vi "GUI_Cameras_v1.2.1.vi"() -> ()   [LabVIEW 2011]
uses:
  <vilib>/Utility/miscctls.llb/LVRectTypeDef.ctl
  <vilib>/vision/NI_Vision_Development_Module.lvlib
panel:
  out "resize":bool
  in  "Tab Control":T1(tab)
  in  "analysis":bool
  out "MaxCounts":dbl(slide) scale=0.0..256.0
  in  "triggerdelay":dbl
  in  "trigger":bool
  in  "save":bool
  in  "exposure":dbl=0.52 caption="Exposure"
  in  "gain":dbl
  in  "shotnumber":i32=354
  out "Centroid":cluster{"X Centroid":sgl, "Y Centroid":sgl} {"Y Centroid" format="%.2f"; "X Centroid" format="%.2f"}
  out "Mean Value":sgl format="%.2f"
  out "Mean Value 2":sgl(graph)
  out "histogram":T2(graph)
  out "lineout":cluster{"x0":sgl, "dx":sgl, "Pixels Line":sgl[]}(graph)
  out "analysis error":errorcluster
  out "top":i16
  out "left":i16
  out "Zoom changed":bool
  out "Zoom old":cluster{"X":sgl, "Y":sgl}
  out "ratio(h)":bool=TRUE
  out "fixsize":bool
  out "Change Ratio":cluster{"X":sgl, "Y":sgl}={"X"=1.6671598, "Y"=0.6151203}
  out "old Panel Bounds":T3={"Left"=105, "Top"=80, "Right"=781, "Bottom"=662}
  out "error (h)":bool
  in  "Main Tap":enum32{"IMAQ", "Network", "Internal", "Array"}(tab)
  out "Image (IMAQ)":T4(plugin-control)
  out "local Port":u16=65401
  out "Remote Host":string="192.168.10.157"
  out "port or service name":u16=65400
  in  "timeout ms (slow resp)":i32=500
  in  "reset":bool
  out "All Devices (h)":string[](array[string])
  out "centroidy":dbl
  out "fast ID (h)":refnum<k16>
  out "slow ID (h)":refnum<k16>
  out "error out":errorcluster
  out "connections (hidden)":variant[](array[variant])=[variant(refnum<k16> refnum), variant(refnum<k16> refnum)]
  in  "time to wait (main loop)":i32=200
  in  "time to wait (TCP)":i32=10
  out "Data String":string="exposure,0.520000\r\ntrigger,off\r\nsave,off\r\ngain,0.000000\r\n"
  in  "send":bool
  in  "localsavingpath":path
  out "centroidy":dbl
  out "Image (array)":u8[][](graph)
  out "Device Name (h)":string="FakeCam1"
  out "stop":bool
  out "error message":string
  out "image connection":bool
  out "data connection ok":bool
  # "Data"
  # "Image"
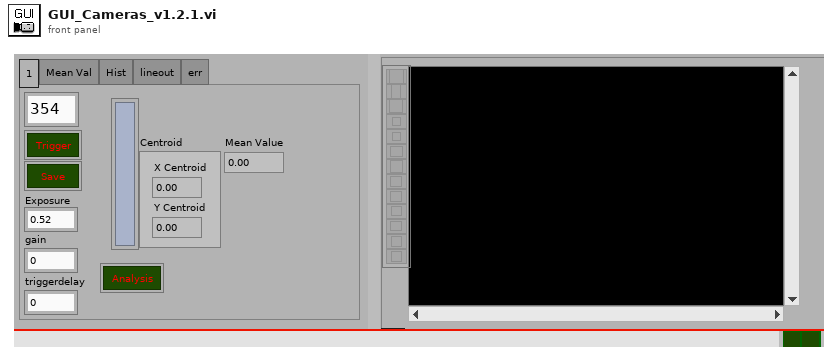
[diagram p1: front panel]
types:
  T1 = enum32{"1", "Mean Val", "Hist", "lineout", "err"}
  T2 = cluster{"Starting Value":sgl, "Incremental Value":sgl, "Histogram":u32[]}
  T3 = typedef "LVRectTypeDef.ctl" = cluster{"Left":i16, "Top":i16, "Right":i16, "Bottom":i16}
  T4 = typedef "IMAQ Image.ctl" = refnum<image>
  T5 = enum16{"Grayscale", "Binary", "Gradient", "Rainbow", "Temperature", "User Defined"}
  T6 = typedef "Image Type" = u32
  T7 = typedef "EventTypDef.ctl" = refnum<user-event>
  T8 = cluster{"Global Rectangle":i32[], "Contours":cluster{"Contour Type":u32, "ROI Type":u32, "Points":i32[]}[]}
  T9 = typedef "IMAQ Line" = cluster{"Start X":i32, "Start Y":i32, "End X":i32, "End Y":i32}
  T10 = typedef "ROI Descriptor" = cluster{"Global Rectangle":i32[], "Contours":cluster{"ID":enum32{"External", "Internal"}, "Type":u32, "Coordinates":i32[]}[]}
  T11 = typedef "LVBoundsTypeDef.ctl" = cluster{"Width":u32, "Height":u32}
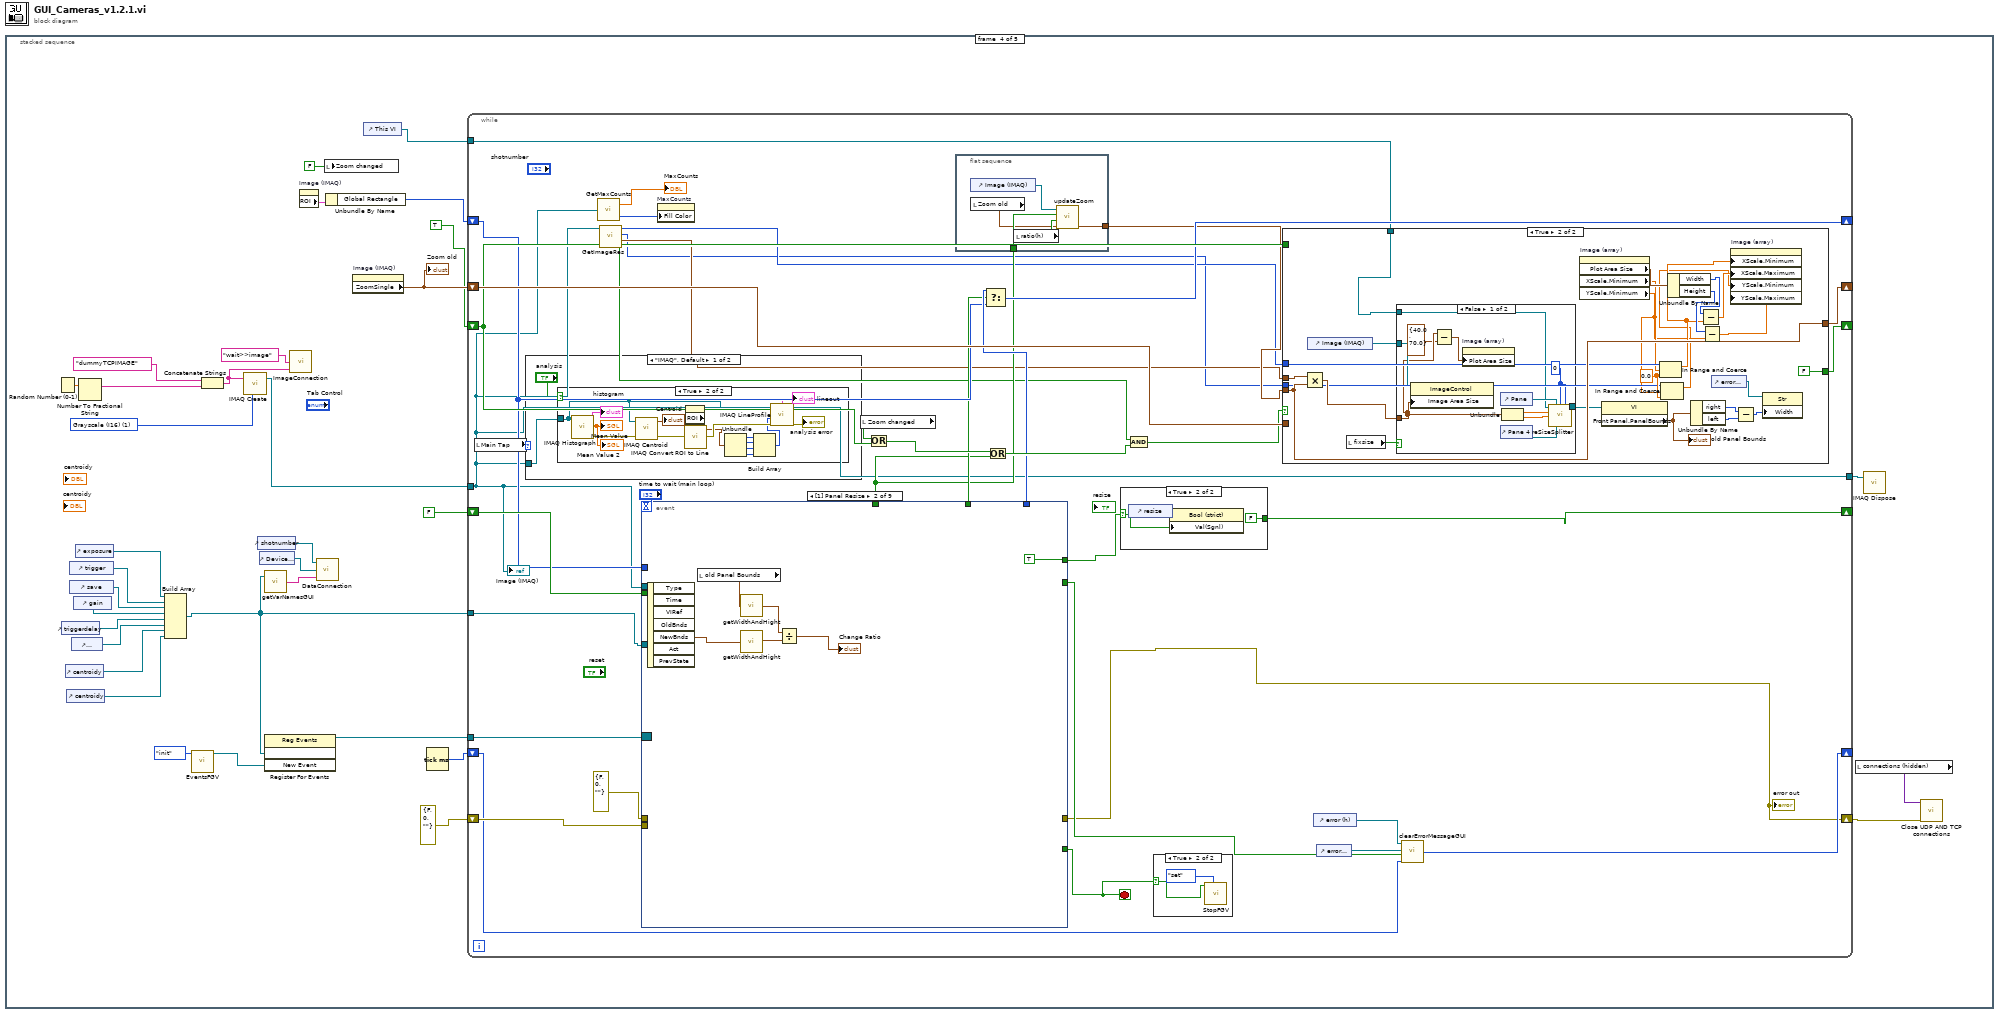
[diagram p0: block diagram]
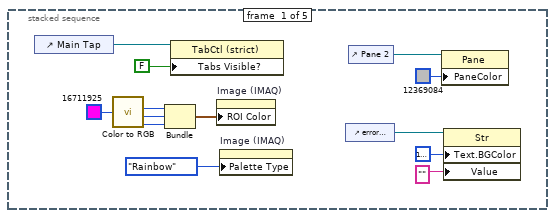
[diagram p2: hidden frame]
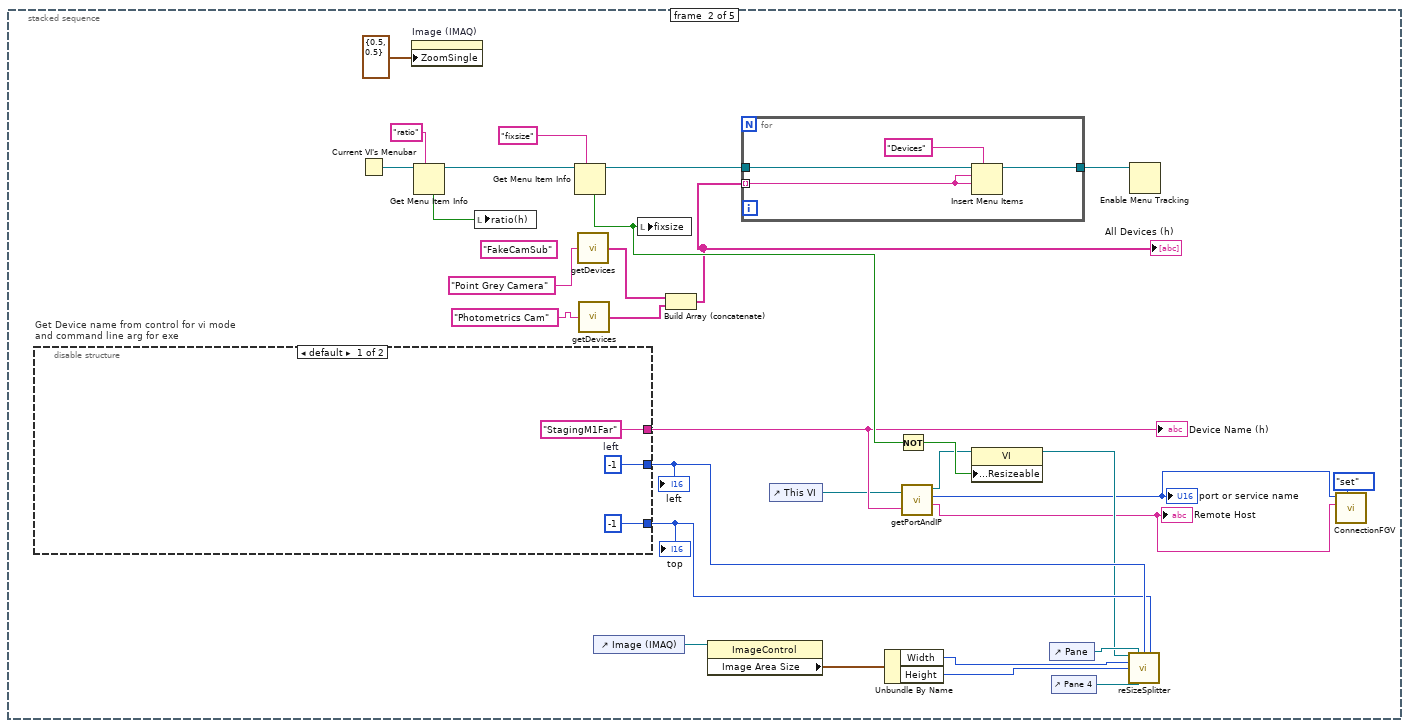
[diagram p3: hidden frame]
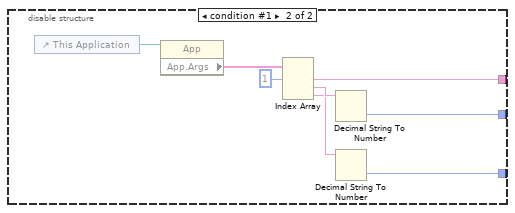
[diagram p4: hidden frame]
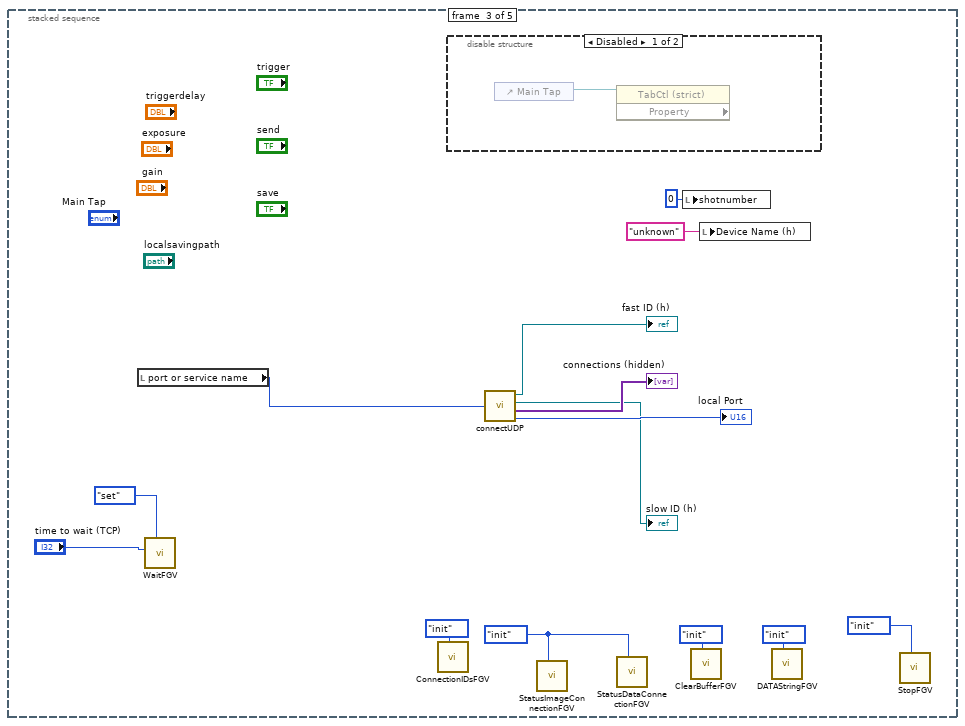
[diagram p5: hidden frame]
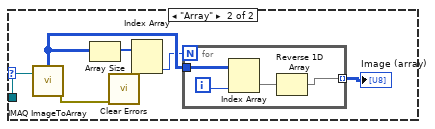
[diagram p10: hidden frame]
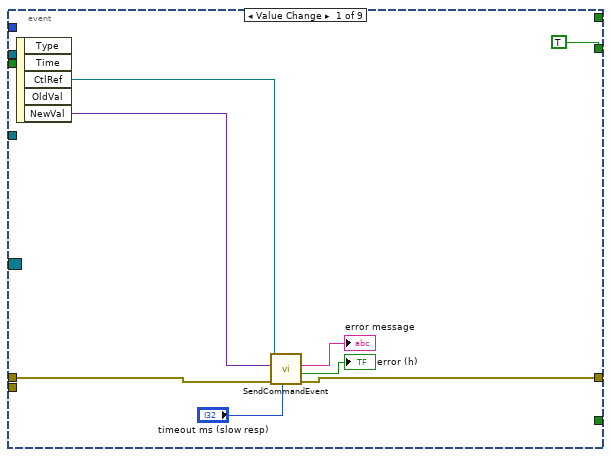
[diagram p13: hidden frame]
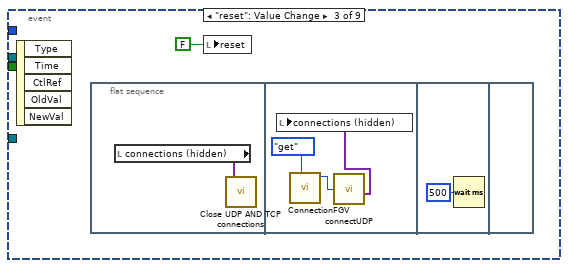
[diagram p14: hidden frame]
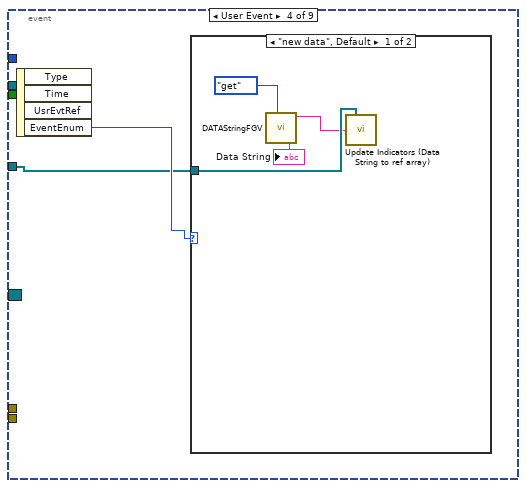
[diagram p15: hidden frame]
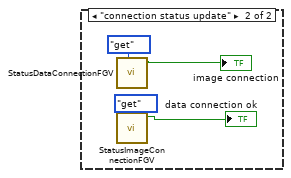
[diagram p16: hidden frame]
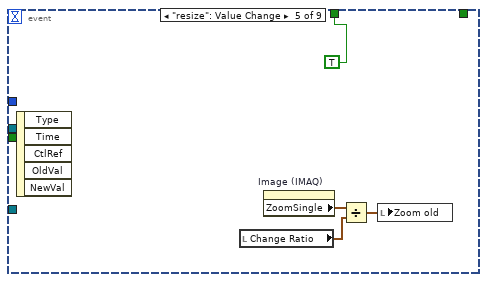
[diagram p17: hidden frame]
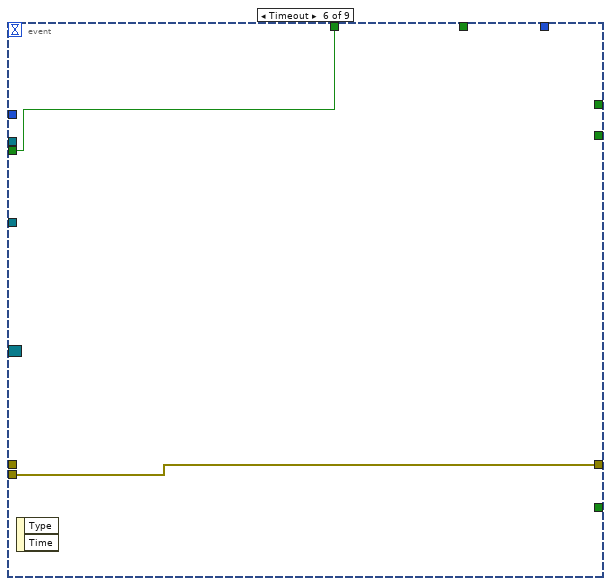
[diagram p18: hidden frame]
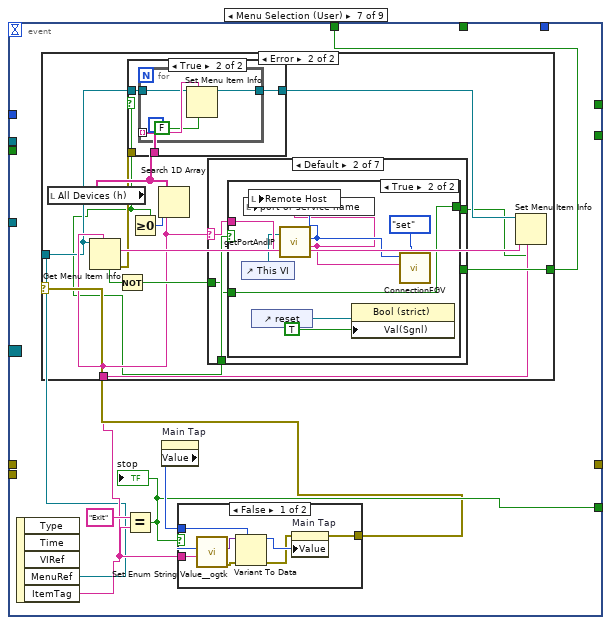
[diagram p19: hidden frame]
diagram:
  n1 = stacked-sequence {
    frame #0 {
      n2 = control-ref of="Main Tap"() -> (w13:refnum<vi>)
      n3 = call <vilib>:"Color to RGB.vi"("Color"=u32 16711925) -> ("R"=w4:u8, "G"=w3:u8, "B"=w2:u8)  [unwired: 1 out]
      n4 = Bundle("R"=w4, "G"=w3, "B"=w2) -> (w1:cluster{"R":u8, "G":u8, "B":u8})  [unwired: 1 in]
      n5 = property class="TabCtl (strict)"(reference=w13, "Tabs Visible?"=FALSE) -> ()  [unwired: 1 in, 2 out]
      n6 = property on="Image (IMAQ)" class="ImageControl"("ROI Color"=w1) -> ()  [unwired: 2 in, 2 out]
      n7 = property on="Image (IMAQ)" class="ImageControl"("Palette Type"=T5."Rainbow" ("Palette:Palette Type")) -> ()  [unwired: 2 in, 2 out]
      n8 = control-ref of="error message"() -> (w10:refnum<vi>)
      n9 = control-ref of="Pane 2"() -> (w8:refnum<vi>)
      n10 = property class="Pane"(reference=w8, "PaneColor"=u32 12369084) -> ()  [unwired: 1 in, 2 out]
      n11 = property class="Str"(reference=w10, "Text.BGColor"=u32 16777238, "Value"="") -> ()  [unwired: 1 in, 2 out]
    }
    frame #1 {
      (unwired) "FakeCamSub" ("Device Class")
      n12 = disable-structure "Get Device name from control for vi mode\nand command line arg for exe" shown="default" {
        disable-tunnel: ["StagingM1Far" ("Device Name for vi mode") w55] -> w25
        disable-tunnel: [w49 w52] -> w32
        disable-tunnel: [i16 -1 ("left") w51] -> w31
        frame condition #0 (active) {
          w49 = i16 -1  # left
        }
        frame condition #1 {
          n13 = control-ref of="This Application"() -> (w58:refnum<vi>)
          n14 = property class="App"(reference=w58) -> ("App.Args"=w57:string[])  [unwired: 1 in, 2 out]
          n15 = Index Array(array=w57, index #1=1 ("index")) -> (element #1=w55:string, element #2=w54:string, element #3=w53:string)  [unwired: 2 in]
          n16 = Decimal String To Number(string=w54) -> (number=w52:i32)  [unwired: 2 in, 1 out]
          n17 = Decimal String To Number(string=w53) -> (number=w51:i32)  [unwired: 2 in, 1 out]
        }
      }
      "Device Name (h)" <- w25
      "left" <- w32
      "top" <- w31
      n18 = Current VI's Menubar() -> (w36:refnum<k9>)
      n19 = property on="Image (IMAQ)" class="ImageControl"("ZoomSingle"=cluster{"X":sgl, "Y":sgl} {"X"=0.5, "Y"=0.5} ("ZoomSingle:All Elements")) -> ()  [unwired: 2 in, 2 out]
      n20 = Get Menu Item Info(7:"ratio" ("item tag"), 11:w36) -> (3:w34:refnum<k9>, 4:w35:bool)  [unwired: 1 in, 5 out]
      n21 = local write "ratio(h)"(w35) -> ()
      n22 = Get Menu Item Info(7:"fixsize" ("item tag"), 11:w34) -> (3:w27:refnum<k9>, 4:w29:bool)  [unwired: 1 in, 5 out]
      n23 = call "getDevices.vi"("Device Class"="Point Grey Camera") -> ("All Devices"=w16:string[])
      n24 = call "getDevices.vi"("Device Class"="Photometrics Cam") -> ("All Devices"=w15:string[])
      n25 = control-ref of="Image (IMAQ)"() -> (w43:refnum<vi>)
      n26 = local write "fixsize"(w29) -> ()
      n27 = Build Array (concatenate)(w16, w15) -> (w14:string[])
      "All Devices (h)" <- w14
      n28 = property class="ImageControl"(reference=w43) -> ("Image Area Size"=w42:cluster{"Width":u32, "Height":u32})  [unwired: 1 in, 2 out]
      n29 = for {
        tunnel: w27 -> [w47]
        tunnel: [w46] -> w26
        tunnel: w14 -> [w44] mode=indexing
        n30 = Insert Menu Items(5:"Devices" ("menu tag"), 7:w44, 8:w44, 9:w47) -> (3:w46:refnum<k9>)  [unwired: 2 in, 2 out]
      }
      n31 = control-ref of="This VI"() -> (w24:refnum<vi>)
      n32 = Unbundle By Name(w42) -> ("Width"=w41:u32, "Height"=w40:u32)
      n33 = Not(x=w29) -> (.not. x?=w30:bool)
      n34 = call "getPortAndIP.vi"("This Vi"=w24, "Device Name"=w25) -> ("reference out"=w23:refnum<vi>, "port or service name"=w20:u16, "Remote Host"=w19:string)  [unwired: 1 in]
      "port or service name" <- w20
      "Remote Host" <- w19
      n35 = property class="VI"(reference=w23, "Front Panel.Resizeable"=w30) -> (reference out=w22:refnum<vi>)  [unwired: 1 in, 1 out]
      n36 = control-ref of="Pane"() -> (w39:refnum<vi>)
      n37 = control-ref of="Pane 4"() -> (w28:refnum<vi>)
      n38 = call "reSizeSplitter.vi"("this vi"=w22, "pane"=w39, "left"=w32, "top"=w31, "Width"=w41, "Height"=w40, "pane2"=w28) -> ()  [unwired: 8 in, 1 out]
      n39 = Enable Menu Tracking(4:w26) -> ()  [unwired: 2 in, 2 out]
      n40 = call "ConnectionFGV.vi"("command"=enum16{"get", "set", "init"}."set", "Remote Host in"=w19, "port or service name in"=w20) -> ()  [unwired: 7 in, 2 out]
    }
    frame #2 {
      w68 = enum16{"get", "set", "init"}."init" ("Command")
      n41 = local read "port or service name"() -> (w70:u16)
      n42 = call "WaitFGV.vi"("Command"=enum16{"get", "set", "init"}."set", "milliseconds to wait"="time to wait (TCP)") -> ()  [unwired: 9 in, 1 out]
      n43 = call "ConnectionIDsFGV.vi"("Command"=enum16{"add", "get", "init"}."init") -> ()  [unwired: 10 in, 1 out]
      n44 = disable-structure shown="Disabled" {
        frame Disabled {
          n45 = control-ref of="Main Tap"() -> (w73:refnum<vi>)
          n46 = property class="TabCtl (strict)" props=[](reference=w73) -> ()  [unwired: 1 in, 3 out]
        }
        frame Enabled {
        }
      }
      n47 = call "connectUDP.vi"("port or service name"=w70) -> ("fast ID (h)"=→"fast ID (h)":refnum<k16>, "slow ID (h)"=→"slow ID (h)":refnum<k16>, "connections (hidden)"=→"connections (hidden)":variant[], "local Port"=→"local Port":u16)
      n48 = call "StatusImageConnectionFGV.vi"("Command"=w68) -> ()  [unwired: 10 in, 1 out]
      n49 = call "StatusDataConnectionFGV.vi"("Command"=w68) -> ()  [unwired: 10 in, 1 out]
      n50 = local write "shotnumber"(0 ("shotnumber")) -> ()
      n51 = call "ClearBufferFGV.vi"("Command"=enum16{"set", "get", "init"}."init") -> ()  [unwired: 10 in, 1 out]
      n52 = local write "Device Name (h)"("unknown" ("Device Name")) -> ()
      n53 = call "DATAStringFGV.vi"("Command"=enum16{"get", "set", "init"}."init") -> ()  [unwired: 10 in, 1 out]
      n54 = call "StopFGV.vi"("Command"=enum16{"set", "get", "init"}."init") -> ()  [unwired: 10 in, 1 out]
    }
    frame #3 {
      w105 = T6 1 items=["Grayscale (U8)", "Grayscale (I16)", "Grayscale (SGL)", "Complex (CSG)", "RGB (U32)", "HSL (U32)", "RGB (U64)", "Grayscale (U16)"] ("Image Type")
      n55 = Random Number (0-1)() -> (number: 0 to 1=w102:dbl)
      n56 = control-ref of="triggerdelay"() -> (w92:refnum<vi>)
      n57 = control-ref of="centroidy"() -> (w86:refnum<vi>)
      n58 = control-ref of="centroidy"() -> (w79:refnum<vi>)
      n59 = control-ref of="trigger"() -> (w96:refnum<vi>)
      n60 = control-ref of="save"() -> (w94:refnum<vi>)
      n61 = control-ref of="localsavingpath"() -> (w87:refnum<vi>)
      n62 = control-ref of="gain"() -> (w93:refnum<vi>)
      n63 = control-ref of="exposure"() -> (w95:refnum<vi>)
      n64 = Number To Fractional String(number=w102) -> (F-format string=w101:string)  [unwired: 3 in]
      n65 = Build Array(w95, w96, w94, w93, w92, w87, w86, w79) -> (w77:refnum<vi>[])
      n66 = call "EventsFGV.vi"("Command"=enum16{"get", "init"}."init") -> ("New Event"=w74:T7)  [unwired: 10 in]
      n67 = Concatenate Strings("dummyTCPIMAGE" ("Image Name"), w101) -> (w99:string)
      n68 = call "IMAQ Create"("Image Name"=w99, "Image Type"=w105) -> ("New Image"=w104:T4)  [unwired: 3 in, 1 out]
      n69 = control-ref of="shotnumber"() -> (w81:refnum<vi>)
      n70 = control-ref of="Device Name (h)"() -> (w80:refnum<vi>)
      n71 = call "getVarNamesGUI.vi"("Array"=w77) -> ("String"=w76:string)  [unwired: 1 in]
      n72 = register-events(w77, w74) -> (reference out=w78:refnum<event-registration>)  [unwired: 2 in, 1 out]
      n73 = call "ImageConnection.vi"("Image Name"=w99, "Image Subscriber list"="wait>>image") -> ()  [unwired: 2 in]
      n74 = property on="Image (IMAQ)" class="ImageControl"() -> ("ROI"=w85:T8)  [unwired: 2 in, 2 out]
      n75 = call "DataConnection.vi"("Subscriber list"=w76, "Device Name (h)"=w80, "shotnumber"=w81) -> ()
      n76 = local write "Zoom changed"(FALSE ("Zoom changed")) -> ()
      n77 = Unbundle By Name(w85) -> ("Global Rectangle"=w84:i32[])
      n78 = property on="Image (IMAQ)" class="ImageControl"() -> ("ZoomSingle"=w91:cluster{"X":sgl, "Y":sgl})  [unwired: 2 in, 2 out]
      "Zoom old" <- w91
      n79 = control-ref of="This VI"() -> (w83:refnum<vi>)
      n80 = Tick Count (ms)() -> (millisecond timer value=w88:u32)
      n81 = while {
        shift-right: [w110] -> w103
        shift-left: errorcluster {"status"=FALSE, "code"=0, "source"=""} ("error out") -> [w143]
        tunnel: w104 -> [w119]
        tunnel: [w119] -> w106
        tunnel: w77 -> [w111]
        shift-right: [w142] -> _
        shift-left: w91 -> [w141]
        shift-right: [w108] -> _
        shift-left: FALSE -> [w140]
        shift-right: [w139] -> _
        shift-left: TRUE -> [w138]
        shift-right: [w134] -> _
        shift-left: w88 -> [w133]
        shift-right: [w128] -> _
        shift-left: w84 -> [w127]
        tunnel: w83 -> [w125]
        tunnel: w78 -> [w112]
        stop <- w113 stop-if-true
        n82 = local read "Main Tap"() -> (w130:enum32{"IMAQ", "Network", "Internal", "Array"})
        n83 = case shown="\"IMAQ\", Default" w130 {
          tunnel: w119 -> [w158 w179]
          frame "IMAQ", Default {
            n84 = case shown="True" "analysis" {
              tunnel: w158 -> [_ w169]
              frame False {
              }
              frame True {
                n85 = call "IMAQ Histograph"("Image"=w169) -> ("error out"=w171:errorcluster, "Mean Value"=→"Mean Value" →"Mean Value 2":sgl, "Histogram Graph"=→"histogram":T2)  [unwired: 7 in, 1 out]
                n86 = call "IMAQ Centroid"("error in (no error)"=w171, "Image"=w169) -> ("error out"=w168:errorcluster, "Centroid"=→"Centroid":cluster{"X Centroid":sgl, "Y Centroid":sgl})  [unwired: 2 in]
                n87 = property on="Image (IMAQ)" class="ImageControl"() -> ("ROI"=w165:T8)  [unwired: 2 in, 2 out]
                n88 = call "IMAQ Convert ROI to Line"("ROI Descriptor"=w165) -> ("Line"=w164:T9)  [unwired: 8 in, 1 out]
                n89 = Unbundle(w164) -> ("Start X"=w163:i32, "Start Y"=w162:i32, "End X"=w161:i32, "End Y"=w160:i32)
                n90 = Build Array(w163, w162, w161, w160) -> (w159:i32[])
                n91 = call "IMAQ LineProfile"("error in (no error)"=w168, "Line Coordinates"=w159, "Image"=w169) -> ("error out"=→"analysis error":errorcluster, "Line Graph"=→"lineout":cluster{"x0":sgl, "dx":sgl, "Pixels Line":sgl[]})  [unwired: 2 in, 2 out]
              }
            }
          }
          frame "Array" {
            n92 = call "IMAQ ImageToArray"("Image"=w179) -> ("error out"=w178:errorcluster, "Image Pixels (U8)"=w175:u8[][])  [unwired: 3 in, 3 out]
            n93 = Array Size(array=w175) -> (size(s)=w177:i32[])
            n94 = call <vilib>:"Clear Errors.vi"("error in (no error)"=w178) -> ()  [unwired: 6 in, 1 out]
            n95 = Index Array(array=w177) -> (element #2=w174:i32)  [unwired: 2 in, 1 out]
            n96 = for {
              N: w174 -> [_]
              tunnel: w175 -> [w183]
              tunnel: [w181] -> w176 mode=indexing
              i -> [w180]
              n97 = Index Array(array=w183, index (col)=w180) -> (element=w182:u8[])  [unwired: 1 in]
              n98 = Reverse 1D Array(array=w182) -> (reversed array=w181:u8[])
            }
            "Image (array)" <- w176
          }
        }
        n99 = call "GetMaxCounts.vi"("New Image"=w119) -> ("Maximal Value"=→"MaxCounts":sgl, "Color"=w121:u32)
        n100 = call "GetImageRes.vi"("Image"=w119) -> ("valid Image"=w117:bool, "Image Area:Size:All Elements"=w118:cluster{"Width":u32, "Height":u32}, "Y Resolution"=w115:i32, "X Resolution"=w116:i32)  [unwired: 7 in]
        n101 = event shown="[1] Panel Resize" {
          selector: w112 -> [_ _ _ _ _ _ _ _ _]
          dyn-events: _ -> [_ _ _ _ _ _ _ _ _]
          timeout: "time to wait (main loop)" -> [_ _ _ _ _ _ _ _ _]
          tunnel: [w228 _ _ _ _ w257 _ _ _] -> w110
          tunnel: errorcluster {"status"=FALSE, "code"=0, "source"=""} ("error out") -> [w230 _ _ _ _ _ _ _ _]
          tunnel: w143 -> [_ _ _ _ _ w257 _ _ _]
          tunnel: [TRUE _ _ _ _ _ _ _ _] -> w131
          tunnel: [_ _ _ _ _ _ w262 _ _] -> w113
          tunnel: [_ _ _ _ TRUE w256 w259 _ _] -> w124
          tunnel: w140 -> [_ _ _ _ _ w256 _ _ _]
          tunnel: [_ TRUE _ _ _ _ _ _ _] -> w109
          tunnel: [_ _ _ _ _ _ _ _ w340] -> w129
          tunnel: w127 -> [_ _ _ _ _ _ _ _ w341]
          tunnel: [_ _ _ _ _ _ _ _ w334] -> w126
          tunnel: w119 -> [_ _ _ _ _ _ _ _ w343]
          tunnel: w111 -> [_ _ _ w243 _ _ _ _ _]
          event Value Change {
            n102 = event-data() -> ("CtlRef"=w225:refnum<vi>, "NewVal"=w224:variant)  [unwired: 1 in, 3 out]
            n103 = call "SendCommandEvent.vi"("timeout ms (slow resp)"="timeout ms (slow resp)", "error out 2"=w230, "NewVal"=w224, "CtlRef"=w225) -> ("error out"=w228:errorcluster, "error (h)"=→"error (h)":bool, "error message"=→"error message":string)  [unwired: 4 in, 1 out]
          }
          event Panel Resize {
            n104 = event-data() -> ("NewBnds"=w236:T3)  [unwired: 1 in, 6 out]
            n105 = local read "old Panel Bounds"() -> (w234:T3)
            n106 = call "getWidthAndHight.vi"("OldBnds"=w234) -> ("output cluster"=w233:cluster{"X":sgl, "Y":sgl})
            n107 = call "getWidthAndHight.vi"("OldBnds"=w236) -> ("output cluster"=w232:cluster{"X":sgl, "Y":sgl})
            n108 = Divide(x=w233, y=w232) -> (x/y=→"Change Ratio":cluster{"X":sgl, "Y":sgl})
          }
          event "reset": Value Change {
            n109 = event-data() -> ()  [unwired: 1 in, 5 out]
            n110 = flat-sequence {
              frame #0 {
                n111 = local read "connections (hidden)"() -> (w238:variant[])
                n112 = call "Close UDP AND TCP connections.vi"("appended array"=w238) -> ()  [unwired: 7 in]
              }
              frame #1 {
                n113 = call "ConnectionFGV.vi"("command"=enum16{"get", "set", "init"}."get") -> ("port or service name out"=w240:u16)  [unwired: 9 in, 1 out]
                n114 = call "connectUDP.vi"("port or service name"=w240) -> ("connections (hidden)"=w239:variant[])  [unwired: 3 out]
                n115 = local write "connections (hidden)"(w239) -> ()
              }
              frame #2 {
                n116 = Wait (ms)(milliseconds to wait=u32 500) -> ()  [unwired: 1 out]
              }
              frame #3 {
              }
            }
            n117 = local write "reset"(FALSE ("reset")) -> ()
          }
          event User Event {
            n118 = event-data() -> ("EventEnum"=w244:enum16{"new data", "connection status update"})  [unwired: 1 in, 3 out]
            n119 = case shown="\"new data\", Default" w244 {
              tunnel: w243 -> [w246 _]
              frame "new data", Default {
                n120 = call "DATAStringFGV.vi"("Command"=enum16{"get", "set", "init"}."get") -> ("Data String out"=w245:string)  [unwired: 10 in]
                "Data String" <- w245
                n121 = call "Update Indicators (Data String to ref array).vi"("Array"=w246, "Data String"=w245) -> ()  [unwired: 12 in, 2 out]
              }
              frame "connection status update" {
                n122 = call "StatusDataConnectionFGV.vi"("Command"=enum16{"get", "set", "init"}."get") -> ("Data Connection out"=→"image connection":bool)  [unwired: 10 in]
                n123 = call "StatusImageConnectionFGV.vi"("Command"=enum16{"get", "set", "init"}."get") -> ("Image Connection out"=→"data connection ok":bool)  [unwired: 10 in]
              }
            }
          }
          event "resize": Value Change {
            n124 = event-data() -> ()  [unwired: 1 in, 5 out]
            n125 = local read "Change Ratio"() -> (w253:cluster{"X":sgl, "Y":sgl})
            n126 = property on="Image (IMAQ)" class="ImageControl"() -> ("ZoomSingle"=w254:cluster{"X":sgl, "Y":sgl})  [unwired: 2 in, 2 out]
            n127 = Divide(x=w254, y=w253) -> (x/y=w252:cluster{"X":sgl, "Y":sgl})
            n128 = local write "Zoom old"(w252) -> ()
          }
          event Timeout {
            n129 = event-data() -> ()  [unwired: 1 in, 2 out]
          }
          event Menu Selection (User) {
            n130 = event-data() -> ("MenuRef"=w258:refnum<k9>, "ItemTag"=w260:string)  [unwired: 1 in, 3 out]
            n131 = Equal?(x="Exit", y=w260) -> (x = y?=w262:bool)
            "stop" <- w262
            n132 = property on="Main Tap" class="TabCtl (strict)"() -> ("Value"=w264:enum32{"IMAQ", "Network", "Internal", "Array"})  [unwired: 2 in, 2 out]
            n133 = case shown="False" w262 {
              tunnel: w264 -> [w323 _]
              tunnel: w260 -> [w322 _]
              tunnel: [w319 errorcluster {"status"=FALSE, "code"=0, "source"=""} ("error out")] -> w261
              frame False {
                n134 = call <userlib>:"Set Enum String Value__ogtk.vi"("String Value"=w322, "Default Enum Value"=w323) -> ("error out"=w321:errorcluster, "Enum"=w325:variant)  [unwired: 8 in]
                n135 = Variant To Data(error in=w321, type=w323, Variant=w325) -> (data=w324:enum32{"IMAQ", "Network", "Internal", "Array"}, error out=w320:errorcluster)
                n136 = property on="Main Tap" class="TabCtl (strict)"(error in=w320, "Value"=w324) -> (error out=w319:errorcluster)  [unwired: 1 in, 1 out]
              }
              frame True {
              }
            }
            n137 = case shown="Error" w261 {
              tunnel: w258 -> [_ w268]
              tunnel: w260 -> [_ w272]
              tunnel: [_ w273] -> w259
              frame No Error {
              }
              frame Error {
                n138 = local read "All Devices (h)"() -> (w270:string[])
                n139 = Get Menu Item Info(7:w272, 11:w268) -> (0:w269:errorcluster, 2:w275:string, 4:w276:bool)  [unwired: 1 in, 4 out]
                n140 = Not(x=w276) -> (.not. x?=w274:bool)
                n141 = Search 1D Array(1D array=w270, element=w272) -> (index of element=w271:i32)  [unwired: 1 in]
                n142 = Greater Or Equal To 0?(x=w271) -> (x >= 0?=w267:bool)
                n143 = case shown="True" w267 {
                  tunnel: w270 -> [_ w280]
                  tunnel: w269 -> [_ _]
                  tunnel: w268 -> [w277 w279]
                  tunnel: [w277 w278] -> w266
                  frame False {
                  }
                  frame True {
                    n144 = for {
                      tunnel: w280 -> [w284] mode=indexing
                      tunnel: w279 -> [w282]
                      tunnel: [w281] -> w278
                      n145 = Set Menu Item Info(6:FALSE ("checked"), 7:w284, 11:w282) -> (3:w281:refnum<k9>)  [unwired: 4 in, 1 out]
                    }
                  }
                }
                n146 = case shown="Default" w272 {
                  selector: w272 -> [_ w290 _ _ w311 _ _]
                  tunnel: w274 -> [w285 w288 w301 _ _ _ w316]
                  tunnel: [_ _ TRUE _ _ _ _] -> w273
                  tunnel: w267 -> [_ w291 _ _ _ _ _]
                  tunnel: [w285 w289 w301 _ _ _ w316] -> w265
                  frame "fixsize" {
                    n147 = control-ref of="This VI"() -> (w287:refnum<vi>)
                    n148 = Not(x=w285) -> (.not. x?=w286:bool)
                    n149 = property class="VI"(reference=w287, "Front Panel.Resizeable"=w286) -> ()  [unwired: 1 in, 2 out]
                    "fixsize" <- w285
                  }
                  frame Default {
                    n150 = case shown="True" w291 {
                      tunnel: w290 -> [_ w299]
                      tunnel: [_ w295] -> w289
                      tunnel: w288 -> [_ w295]
                      frame False {
                      }
                      frame True {
                        n151 = control-ref of="This VI"() -> (w298:refnum<vi>)
                        n152 = control-ref of="reset"() -> (w297:refnum<vi>)
                        n153 = call "getPortAndIP.vi"("This Vi"=w298, "Device Name"=w299) -> ("port or service name"=w293:u16, "Remote Host"=w292:string)  [unwired: 1 in, 1 out]
                        n154 = local write "port or service name"(w293) -> ()
                        n155 = local write "Remote Host"(w292) -> ()
                        n156 = property class="Bool (strict)"(reference=w297, "Val(Sgnl)"=TRUE ("Value (Signaling)")) -> ()  [unwired: 1 in, 2 out]
                        n157 = call "ConnectionFGV.vi"("command"=enum16{"get", "set", "init"}."set", "Remote Host in"=w292, "port or service name in"=w293) -> ()  [unwired: 7 in, 2 out]
                      }
                    }
                  }
                  frame "ratio" {
                    n158 = property on="Image (IMAQ)" class="ImageControl"() -> ("ZoomSingle"=w300:cluster{"X":sgl, "Y":sgl})  [unwired: 2 in, 2 out]
                    n159 = local write "Zoom old"(w300) -> ()
                    "ratio(h)" <- w301
                  }
                  frame "Local Saving Path" {
                    n160 = control-ref of="localsavingpath"() -> (w303:refnum<vi>)
                    n161 = property class="Path"(reference=w303) -> (reference out=w306:refnum<vi>, "Value"=w307:path)  [unwired: 1 in, 1 out]
                    n162 = call "changePath.vi"("Local Saving in (h)"=w307) -> ("change (h)"=w305:bool, "Local Saving out (h)"=w304:path)  [unwired: 9 in]
                    n163 = case shown="True" w305 {
                      tunnel: w306 -> [_ w309]
                      tunnel: w304 -> [_ w308]
                      frame False {
                      }
                      frame True {
                        n164 = property class="Path"(reference=w309, "Val(Sgnl)"=w308) -> ()  [unwired: 1 in, 2 out]
                      }
                    }
                  }
                  frame "Binary", "Gradient", "Grayscale", "Rainbow", "Temperature" {
                    n165 = Scan From String(input string=w311, default 1=T5."Grayscale" ("Palette:Palette Type")) -> (output 1=w310:T5)  [unwired: 3 in, 3 out]
                    n166 = property on="Image (IMAQ)" class="ImageControl"("Palette Type"=w310) -> ()  [unwired: 2 in, 2 out]
                  }
                  frame "reset" {
                    n167 = control-ref of="reset"() -> (w314:refnum<vi>)
                    n168 = property class="Bool (strict)"(reference=w314, "Val(Sgnl)"=TRUE ("Value (Signaling)")) -> ()  [unwired: 1 in, 2 out]
                  }
                  frame "clear" {
                    n169 = control-ref of="reset"() -> (w318:refnum<vi>)
                    n170 = call "ClearBufferFGV.vi"("Command"=enum16{"set", "get", "init"}."set", "clear buffer"=w316) -> ()  [unwired: 9 in, 1 out]
                    n171 = property class="Bool (strict)"(reference=w318, "Val(Sgnl)"=TRUE ("Value (Signaling)")) -> ()  [unwired: 1 in, 2 out]
                  }
                }
                n172 = Set Menu Item Info(6:w265, 7:w272, 10:w275, 11:w266) -> ()  [unwired: 3 in, 2 out]
              }
            }
          }
          event "time to wait (TCP)": Value Change {
            n173 = event-data() -> ("NewVal"=w328:i32)  [unwired: 1 in, 4 out]
            n174 = call "WaitFGV.vi"("Command"=enum16{"get", "set", "init"}."set", "milliseconds to wait"=w328) -> ()  [unwired: 9 in, 1 out]
          }
          event "Image (IMAQ)": Mouse Up {
            n175 = event-data() -> ()  [unwired: 1 in, 5 out]
            n176 = property on="Image (IMAQ)" class="ImageControl"() -> ("ROI"=w342:T8)  [unwired: 2 in, 2 out]
            n177 = Unbundle By Name(w342) -> ("Global Rectangle"=w340:i32[])
            n178 = Not Equal?(x=w341, y=w340) -> (x != y?=w344:bool[])
            n179 = property on="Image (IMAQ)" class="ImageControl"() -> ("ZoomSingle"=w329:cluster{"X":sgl, "Y":sgl})  [unwired: 2 in, 2 out]
            n180 = local read "Zoom old"() -> (w331:cluster{"X":sgl, "Y":sgl})
            n181 = Empty Array?(array=w341) -> (empty?=w337:bool)
            n182 = Empty Array?(array=w340) -> (empty?=w339:bool)
            n183 = Or Array Elements(Boolean array=w344) -> (logical OR=w335:bool)
            n184 = Not(x=w339) -> (.not. x?=w338:bool)
            n185 = And(x=w337, y=w338) -> (x .and. y?=w336:bool)
            n186 = Unbundle By Name(w329) -> ("X"=w332:sgl)
            n187 = Unbundle By Name(w331) -> ("X"=w333:sgl)
            n188 = Not Equal?(x=w332, y=w333) -> (x != y?=w330:bool)
            "Zoom changed" <- w330
            n189 = Or(x=w335, y=w336) -> (x .or. y?=w334:bool)
            n190 = case shown="True" w334 {
              tunnel: w343 -> [_ _]
              tunnel: w342 -> [_ w347]
              frame False {
              }
              frame True {
                n191 = call "ROI thickener.vi"("ROI Descriptor in"=w347) -> ("ROI Descriptor out"=w346:T10)  [unwired: 1 in, 1 out]
                n192 = property on="Image (IMAQ)" class="ImageControl"("ROI"=w346) -> ()  [unwired: 2 in, 2 out]
              }
            }
            n193 = case shown="True" w330 {
              tunnel: w329 -> [_ w345]
              frame False {
              }
              frame True {
                n194 = local write "Zoom old"(w345) -> ()
              }
            }
          }
        }
        "error out" <- w110
        n195 = property on="MaxCounts" class="Slide (strict)"("Fill Color"=w121) -> ()  [unwired: 2 in, 2 out]
        n196 = local read "Zoom changed"() -> (w120:bool)
        n197 = Or(x=w120, y=w138) -> (x .or. y?=w137:bool)
        n198 = flat-sequence {
          tunnel: w124 -> [w155]
          tunnel: [w152] -> w123
          frame #0 {
            n199 = control-ref of="Image (IMAQ)"() -> (w156:refnum<vi>)
            n200 = local read "Zoom old"() -> (w153:cluster{"X":sgl, "Y":sgl})
            n201 = local read "ratio(h)"() -> (w154:bool)
            n202 = call "updateZoom.vi"("Zoom old"=w153, "ratio(h)"=w154, "update Zoom"=w155, "imageRef"=w156) -> ("Zoom out"=w152:cluster{"X":sgl, "Y":sgl})  [unwired: 7 in]
          }
        }
        n203 = Select(t=w129, s=w126, f=w127) -> (s? t:f=w128:i32[])
        n204 = Or(x=w137, y=w124) -> (x .or. y?=w135:bool)
        n205 = case shown="True" w109 {
          selector: w109 -> [w146 w148]
          tunnel: [w146 FALSE] -> w108
          frame False {
          }
          frame True {
            n206 = control-ref of="resize"() -> (w149:refnum<vi>)
            n207 = property class="Bool (strict)"(reference=w149, "Val(Sgnl)"=w148) -> ()  [unwired: 1 in, 2 out]
          }
        }
        n208 = And(x=w117, y=w135) -> (x .and. y?=w136:bool)
        n209 = case shown="True" w113 {
          selector: w113 -> [_ w150]
          frame False {
          }
          frame True {
            n210 = call "StopFGV.vi"("Command"=enum16{"set", "get", "init"}."set", "Stop"=w150) -> ()  [unwired: 9 in, 1 out]
          }
        }
        n211 = case shown="True" w136 {
          tunnel: w123 -> [_ w209]
          tunnel: [w185 w209] -> w142
          tunnel: w141 -> [w185 _]
          tunnel: w118 -> [_ w210]
          tunnel: w138 -> [w184 _]
          tunnel: [w184 FALSE] -> w139
          tunnel: w116 -> [_ w194]
          tunnel: w115 -> [_ w190]
          tunnel: w125 -> [_ w187]
          frame False {
          }
          frame True {
            w191 = 0.0 ("lower limit")
            n212 = Multiply(x=w210, y=w209) -> (x*y=w208:cluster{sgl, sgl})
            n213 = control-ref of="Image (IMAQ)"() -> (w199:refnum<vi>)
            n214 = local read "fixsize"() -> (w200:bool)
            n215 = case shown="False" w200 {
              tunnel: w208 -> [w214 _]
              tunnel: w187 -> [w218 w222]
              tunnel: [w217 w222] -> w206
              tunnel: w199 -> [w216 _]
              frame False {
                w211 = i16 0 ("left")
                n216 = property class="ImageControl"(reference=w216, "Image Area Size"=w214) -> ()  [unwired: 1 in, 2 out]
                n217 = Subtract(x=w214, y=cluster{sgl, sgl} {40.0, 70.0}) -> (x-y=w213:cluster{sgl, sgl})
                n218 = property on="Image (array)" class="IntGraph (strict)"("Plot Area Size"=w213) -> ()  [unwired: 2 in, 2 out]
                n219 = control-ref of="Pane"() -> (w219:refnum<vi>)
                n220 = control-ref of="Pane 4"() -> (w215:refnum<vi>)
                n221 = Unbundle(w214) -> (w220:sgl, w221:sgl)
                n222 = call "reSizeSplitter.vi"("this vi"=w218, "pane"=w219, "left"=w211, "top"=w211, "Width"=w220, "Height"=w221, "pane2"=w215) -> ("reference out"=w217:refnum<vi>)  [unwired: 8 in]
              }
              frame True {
              }
            }
            n223 = property on="Image (array)" class="IntGraph (strict)"() -> ("Plot Area Size"=w198:T11, "XScale.Minimum"=w192:dbl, "YScale.Minimum"=w189:dbl)  [unwired: 2 in, 2 out]
            n224 = property class="VI"(reference=w206) -> ("Front Panel.PanelBounds"=w205:T3)  [unwired: 1 in, 2 out]
            "old Panel Bounds" <- w205
            n225 = In Range and Coerce(upper limit=w194, x=w192, lower limit=w191) -> (coerced(x)=w193:dbl)  [unwired: 1 out]
            n226 = In Range and Coerce(upper limit=w190, x=w189, lower limit=w191) -> (coerced(x)=w188:dbl)  [unwired: 1 out]
            n227 = Unbundle By Name(w198) -> ("Width"=w197:u32, "Height"=w195:u32)
            n228 = Unbundle By Name(w205) -> ("right"=w204:i16, "left"=w203:i16)
            n229 = Subtract(x=w197, y=w193) -> (x-y=w196:dbl)
            n230 = Subtract(x=w195, y=w189) -> (x-y=w186:dbl)
            n231 = control-ref of="error message"() -> (w207:refnum<vi>)
            n232 = property on="Image (array)" class="IntGraph (strict)"("XScale.Minimum"=w193, "XScale.Maximum"=w196, "YScale.Minimum"=w188, "YScale.Maximum"=w186) -> ()  [unwired: 2 in, 2 out]
            n233 = Subtract(x=w204, y=w203) -> (x-y=w202:i16)
            n234 = property class="Str"(reference=w207, "Width"=w202) -> ()  [unwired: 1 in, 2 out]
          }
        }
        n235 = control-ref of="error (h)"() -> (w114:refnum<vi>)
        n236 = control-ref of="error message"() -> (w132:refnum<vi>)
        n237 = call "clearErrorMessageGUI.vi"("millisecond timer value"=w133, "Boolean"=w131, "error message"=w132, "reference"=w114) -> ("millisecond timer value 2"=w134:u32)
        "Image (IMAQ)" <- w119
      }
      n238 = local read "connections (hidden)"() -> (w98:variant[])
      n239 = call "IMAQ Dispose"("Image"=w106) -> ()  [unwired: 5 in, 1 out]
      n240 = call "Close UDP AND TCP connections.vi"("error in"=w103, "appended array"=w98) -> ()  [unwired: 6 in]
    }
    frame #4 {
      n241 = flat-sequence {
        frame #0 {
          n242 = Wait (ms)(milliseconds to wait=u32 0) -> ()  [unwired: 1 out]
        }
        frame #1 {
          n243 = local write "stop"(FALSE ("stop")) -> ()
        }
        frame #2 {
          n244 = control-ref of="This VI"() -> (w355:refnum<vi>)
          n245 = case shown="True" FALSE {
            tunnel: w355 -> [w356 w359]
            tunnel: [w356 w357] -> w354
            frame False {
            }
            frame True {
              n246 = property class="VI" props=["Front Panel.Open"](reference=w359) -> (reference out=w358:refnum<vi>)  [unwired: 1 in, 2 out]
              n247 = invoke class="VI" method="FP.Close"(reference=w358) -> (reference out=w357:refnum<vi>)  [unwired: 2 in, 2 out]
            }
          }
          n248 = Close Reference(reference=w354) -> ()  [unwired: 1 in, 1 out]
        }
      }
      n249 = control-ref of="Main  Control"() -> (w349:refnum<vi>)
      n250 = property class="TabCtl (strict)"(reference=w349, "Tabs Visible?"=TRUE) -> ()  [unwired: 1 in, 2 out]
      n251 = property class="TabCtl (strict)"(reference=w349, "Tab Location"=enum32{"Top", "Bottom", "Left", "Right"}."Bottom") -> ()  [unwired: 1 in, 2 out]
    }
  }
